vi "AuxReadThresholdsFromCfg.vi"(11 "configuration file path":path=path "C:/Users/labadmin/Documents/Jarvis/config/parameter_config.ini") -> (3 "threshholds":cluster{"t1 pmt":i32, "t1 camera":i32})   [LabVIEW 2019]
uses:
  <vilib>/Utility/config.llb/Read Key (I32).vi
  <vilib>/Utility/config.llb/NI_LVConfig.lvlib
panel:
  out "t1 pmt":i32
  out "t1 cam":i32
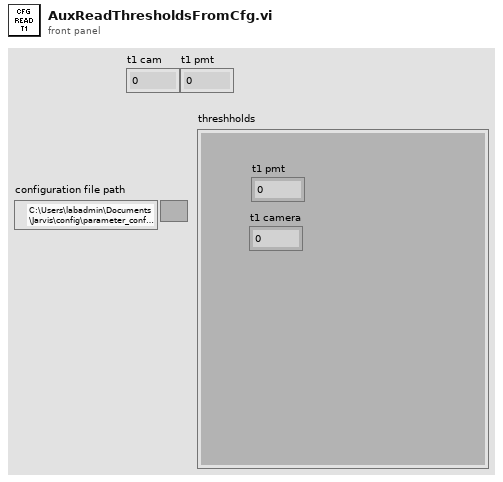
[diagram p1: front panel]
types:
  T1 = typedef "NI_LVConfig.lvlib/Config Data RefNum.ctl" = refnum<k1>
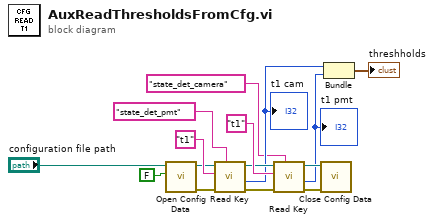
[diagram p0: block diagram]
diagram:
  n1 = call <vilib>:"Open Config Data.vi"("create file if necessary (T)"=FALSE, "configuration file path"="configuration file path") -> ("error out"=w11:errorcluster, "refnum"=w12:T1)  [unwired: 7 in, 1 out]
  n2 = call-poly <vilib>:"Read Key.vi"("section"="state_det_pmt", "error in (no error)"=w11, "key"="t1", "refnum"=w12) -> ("error out"=w9:errorcluster, "value"=w7:i32, "refnum out"=w8:T1)  [unwired: 4 in, 1 out]
  "t1 cam" <- w7
  n3 = call-poly <vilib>:"Read Key.vi"("section"="state_det_camera", "error in (no error)"=w9, "key"="t1", "refnum"=w8) -> ("error out"=w5:errorcluster, "value"=w4:i32, "refnum out"=w6:T1)  [unwired: 4 in, 1 out]
  "t1 pmt" <- w4
  n4 = call <vilib>:"Close Config Data.vi"("error in (no error)"=w5, "refnum"=w6) -> ()  [unwired: 8 in, 2 out]
  n5 = Bundle("value"=w7, "value"=w4) -> (→"threshholds":cluster{"value":i32, "value":i32})  [unwired: 1 in]
